vi "Reallocate_memory.vi"(0 ".NET Refnum in":refnum<k24>, 5 "s32Width":i32, 7 "s32Height":i32, 9 "Bits/Pixel in":i32, 11 "error in (no error)":errorcluster) -> (4 ".NET Refnum Out":refnum<k24>, 15 "error out":errorcluster)   [LabVIEW 2021]
uses:
  C:/Program Files/Thorlabs/Scientific Imaging/ThorCam/uc480DotNet.dll
  Program Files/Thorlabs/Scientific Imaging/ThorCam/uc480DotNet.dll
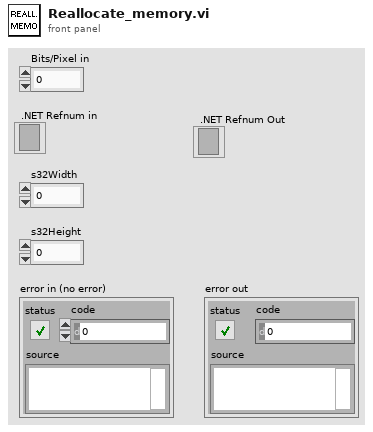
[diagram p1: front panel]
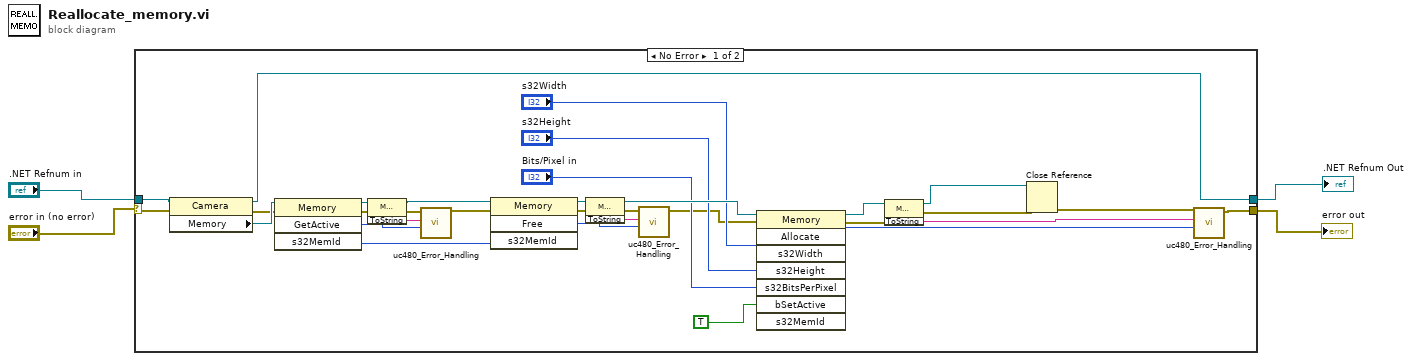
[diagram p0: block diagram]
diagram:
  n1 = case shown="No Error" "error in (no error)" {
    selector: "error in (no error)" -> [w7 w38]
    tunnel: [w27 w38] -> w4
    tunnel: ".NET Refnum in" -> [w6 w37]
    tunnel: [w5 w37] -> w1
    frame No Error {
      n2 = property class="Camera"(reference=w6, error in=w7) -> (reference out=w5:refnum<k24>, error out=w25:errorcluster, "Memory"=w32:refnum<k24>)
      n3 = invoke class="Memory" method="GetActive"(reference=w32, error in=w25) -> (reference out=w20:refnum<k24>, error out=w21:errorcluster, "GetActive"=w22:i32, "s32MemId"=w23:i32)  [unwired: 2 in]
      n4 = invoke class="Memory" method="ToString"(reference=w20, error in=w21) -> (reference out=w33:refnum<k24>, error out=w19:errorcluster, "ToString"=w18:string)  [unwired: 1 in]
      n5 = call "uc480_Error_Handling.vi"("Error Code"=w22, "Error String"=w18, "Error In"=w19) -> ("Error Out"=w24:errorcluster)  [unwired: 8 in]
      n6 = invoke class="Memory" method="Free"(reference=w33, error in=w24, "s32MemId"=w23) -> (reference out=w15:refnum<k24>, error out=w16:errorcluster, "Free"=w17:i32)  [unwired: 1 in, 1 out]
      n7 = invoke class="Memory" method="ToString"(reference=w15, error in=w16) -> (reference out=w36:refnum<k24>, error out=w14:errorcluster, "ToString"=w13:string)  [unwired: 1 in]
      n8 = call "uc480_Error_Handling.vi"("Error Code"=w17, "Error String"=w13, "Error In"=w14) -> ("Error Out"=w26:errorcluster)  [unwired: 8 in]
      n9 = invoke class="Memory" method="Allocate"(reference=w36, error in=w26, "s32Width"="s32Width", "s32Height"="s32Height", "s32BitsPerPixel"="Bits/Pixel in", "bSetActive"=TRUE) -> (reference out=w9:refnum<k24>, error out=w10:errorcluster, "Allocate"=w11:i32)  [unwired: 2 in, 5 out]
      n10 = invoke class="Memory" method="ToString"(reference=w9, error in=w10) -> (reference out=w35:refnum<k24>, error out=w34:errorcluster, "ToString"=w8:string)  [unwired: 1 in]
      n11 = Close Reference(reference=w35, error in (no error)=w34) -> (error out=w31:errorcluster)
      n12 = call "uc480_Error_Handling.vi"("Error Code"=w11, "Error String"=w8, "Error In"=w31) -> ("Error Out"=w27:errorcluster)  [unwired: 8 in]
    }
    frame Error {
    }
  }
  "error out" <- w4
  ".NET Refnum Out" <- w1
